vi "sc5511a_search_devices.vi"(5 "error in (no error)":errorcluster) -> (15 "Number of Devices":i32, 16 "Device SN":string[](array[string]), 19 "error out":errorcluster)   [LabVIEW 2010]
uses:
  sc5511a.dll
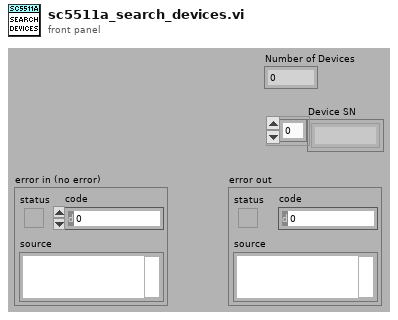
[diagram p1: front panel]
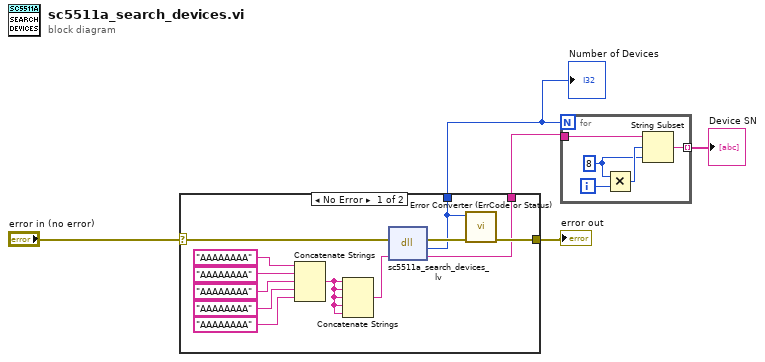
[diagram p0: block diagram]
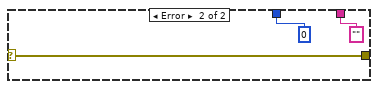
[diagram p2: hidden frame]
diagram:
  n1 = case shown="No Error" "error in (no error)" {
    selector: "error in (no error)" -> [w6 w18]
    tunnel: [w17 w18] -> w4
    tunnel: [w15 "" ("list")] -> w3
    tunnel: [w14 0 ("return type")] -> w2
    frame No Error {
      n2 = Concatenate Strings("AAAAAAAA" ("list"), "AAAAAAAA" ("list"), "AAAAAAAA" ("list"), "AAAAAAAA" ("list"), "AAAAAAAA" ("list")) -> (w7:string)
      n3 = Concatenate Strings(w7, w7, w7, w7, w7) -> (w8:string)
      n4 = dll-call lib="sc5511a.dll" fn="sc5511a_search_devices_lv"(error in=w6, "list"=w8) -> (error out=w16:errorcluster, "return type"=w14:i32, "list"=w15:string)  [unwired: 2 in, 1 out]
      n5 = call "Error Converter (ErrCode or Status).vi"("error in (no error)"=w16, "error code"=w14) -> ("error out"=w17:errorcluster)  [unwired: 9 in]
    }
    frame Error {
    }
  }
  "Number of Devices" <- w2
  "error out" <- w4
  n6 = for {
    N: w2 -> [_]
    tunnel: w3 -> [w22]
    tunnel: [w21] -> w5 mode=indexing
    i -> [w25]
    w23 = 8 ("x")
    n7 = Multiply(x=w23, y=w25) -> (x*y=w24:i32)
    n8 = String Subset(string=w22, offset (0)=w24, length (rest)=w23) -> (substring=w21:string)
  }
  "Device SN" <- w5
